vi "Test_ParseErrorsFromAnswer.vi"() -> (0 "error string (if existing)":string, 1 "error string (if existing) 2":string, 2 "error string (if existing) 3":string, 3 "error string (if existing) 4":string, 4 "error string (if existing) 5":string, 5 "error string (if existing) 6":string, 20 "error out 1":errorcluster, 21 "error out 2":errorcluster, 22 "error out 3":errorcluster, 23 "error out 4":errorcluster, 24 "error out 5":errorcluster, 25 "error out 6":errorcluster)   [LabVIEW 2023]
uses:
  <vilib>/addons/_JKI Toolkits/Caraya/classes/Assert/Assert Error.vi
  <vilib>/addons/_JKI Toolkits/Caraya/classes/Assert/Assert Not Error.vi
  <vilib>/addons/_JKI Toolkits/Caraya/classes/Assert/Assert Equal Value and Type_Variant.vi
  <vilib>/addons/_JKI Toolkits/Caraya/classes/Test/Test.lvclass
  <vilib>/addons/_JKI Toolkits/Caraya/classes/Assert/Assert.lvclass
  Classes/Communicator/Communicator.lvclass
panel:
  out "key found? 6":bool
  out "key found? 5":bool
  out "key found? 4":bool
  out "key found? 3":bool
  out "key found? 2":bool
  out "key found?":bool
  # "Connector Pane"
  # "Locals"
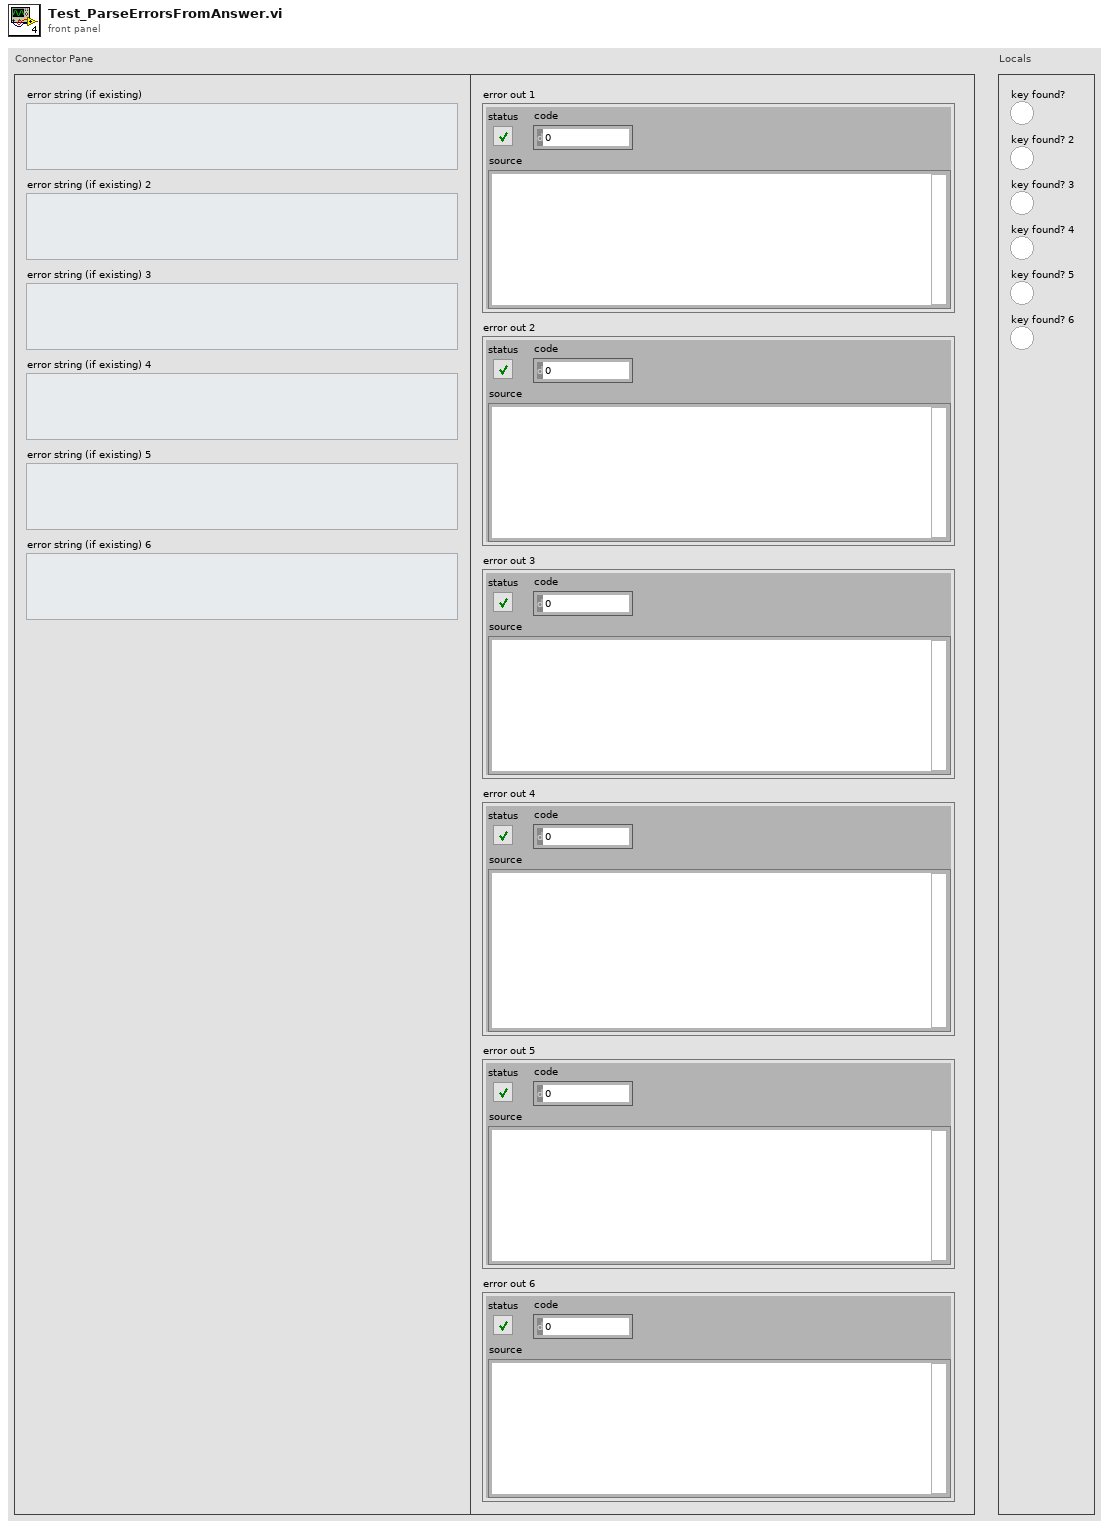
[diagram p1: front panel]
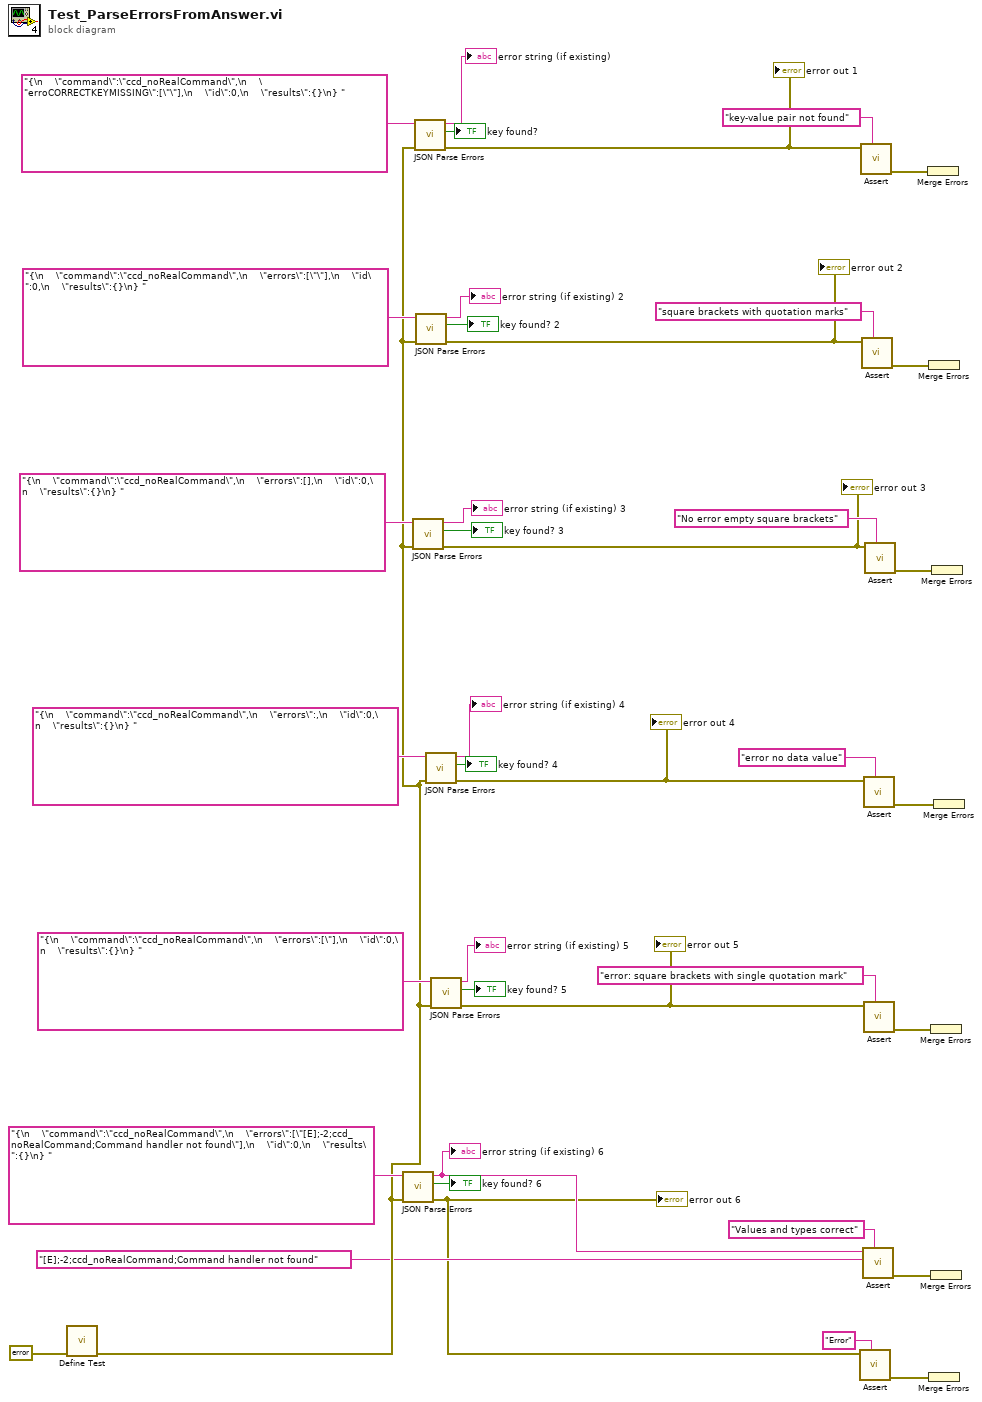
[diagram p0: block diagram]
diagram:
  n1 = call <vilib>:"Define Test.vi"("error in (no error)"=errorcluster {"status"=FALSE, "code"=0, "source"=""}) -> ("error out"=w4:errorcluster)  [unwired: 9 in, 1 out]
  n2 = call "JSON Parse Errors.vi"("error in (no error)"=w4, "JSON command"="{\n    \"command\":\"ccd_noRealCommand\",\n    \"errors\":[\"[E];-2;ccd_noRealCommand;Command handler not found\"],\n    \"id\":0,\n    \"results\":{}\n} ") -> ("error out"=w1:errorcluster, "key found?"=→"key found? 6":bool, "error string (if existing)"=w3:string)  [unwired: 7 in]
  "error string (if existing) 6" <- w3
  "error out 6" <- w1
  n3 = call "JSON Parse Errors.vi"("error in (no error)"=w4, "JSON command"="{\n    \"command\":\"ccd_noRealCommand\",\n    \"errors\":[],\n    \"id\":0,\n    \"results\":{}\n} ") -> ("error out"=w33:errorcluster, "key found?"=→"key found? 3":bool, "error string (if existing)"=→"error string (if existing) 3":string)  [unwired: 7 in]
  "error out 3" <- w33
  n4 = call "JSON Parse Errors.vi"("error in (no error)"=w4, "JSON command"="{\n    \"command\":\"ccd_noRealCommand\",\n    \"erroCORRECTKEYMISSING\":[\"\"],\n    \"id\":0,\n    \"results\":{}\n} ") -> ("error out"=w39:errorcluster, "key found?"=→"key found?":bool, "error string (if existing)"=→"error string (if existing)":string)  [unwired: 7 in]
  "error out 1" <- w39
  n5 = call "JSON Parse Errors.vi"("error in (no error)"=w4, "JSON command"="{\n    \"command\":\"ccd_noRealCommand\",\n    \"errors\":[\"\"],\n    \"id\":0,\n    \"results\":{}\n} ") -> ("error out"=w29:errorcluster, "key found?"=→"key found? 2":bool, "error string (if existing)"=→"error string (if existing) 2":string)  [unwired: 7 in]
  "error out 2" <- w29
  n6 = call "JSON Parse Errors.vi"("error in (no error)"=w4, "JSON command"="{\n    \"command\":\"ccd_noRealCommand\",\n    \"errors\":,\n    \"id\":0,\n    \"results\":{}\n} ") -> ("error out"=w24:errorcluster, "key found?"=→"key found? 4":bool, "error string (if existing)"=→"error string (if existing) 4":string)  [unwired: 7 in]
  "error out 4" <- w24
  n7 = call "JSON Parse Errors.vi"("error in (no error)"=w4, "JSON command"="{\n    \"command\":\"ccd_noRealCommand\",\n    \"errors\":[\"],\n    \"id\":0,\n    \"results\":{}\n} ") -> ("error out"=w21:errorcluster, "key found?"=→"key found? 5":bool, "error string (if existing)"=→"error string (if existing) 5":string)  [unwired: 7 in]
  "error out 5" <- w21
  n8 = call-poly <vilib>:"Assert.vi"("Label"="Error" ("Label (VI Title)"), "Error?"=w1) -> ("error out"=w9:errorcluster)  [unwired: 8 in, 1 out]
  n9 = call-poly <vilib>:"Assert.vi"("Label"="key-value pair not found" ("Label (VI Title)"), "Error?"=w39) -> ("error out"=w38:errorcluster)  [unwired: 8 in, 1 out]
  n10 = call-poly <vilib>:"Assert.vi"("Label"="square brackets with quotation marks" ("Label (VI Title)"), "Error?"=w29) -> ("error out"=w28:errorcluster)  [unwired: 8 in, 1 out]
  n11 = call-poly <vilib>:"Assert.vi"("Label"="Values and types correct" ("Label (VI Title)"), "Y"="[E];-2;ccd_noRealCommand;Command handler not found" ("error string (if existing) 7"), "X"=w3) -> ("error out"=w7:errorcluster)  [unwired: 7 in, 1 out]
  n12 = call-poly <vilib>:"Assert.vi"("Label"="error no data value" ("Label (VI Title)"), "Error?"=w24) -> ("error out"=w25:errorcluster)  [unwired: 8 in, 1 out]
  n13 = call-poly <vilib>:"Assert.vi"("Label"="error: square brackets with single quotation mark" ("Label (VI Title)"), "Error?"=w21) -> ("error out"=w20:errorcluster)  [unwired: 8 in, 1 out]
  n14 = call-poly <vilib>:"Assert.vi"("Label"="No error empty square brackets" ("Label (VI Title)"), "Not Error?"=w33) -> ("error out"=w32:errorcluster)  [unwired: 8 in, 1 out]
  n15 = Merge Errors(w38) -> ()  [unwired: 1 out]
  n16 = Merge Errors(w28) -> ()  [unwired: 1 out]
  n17 = Merge Errors(w9) -> ()  [unwired: 1 out]
  n18 = Merge Errors(w20) -> ()  [unwired: 1 out]
  n19 = Merge Errors(w7) -> ()  [unwired: 1 out]
  n20 = Merge Errors(w32) -> ()  [unwired: 1 out]
  n21 = Merge Errors(w25) -> ()  [unwired: 1 out]
